vi "Set Begin.vi"(8 "error in (no error)":errorcluster, 10 "Begin":refnum<class "Data.lvclass">, 11 "Range in":refnum<class "Range.lvclass">) -> (0 "error out":errorcluster, 3 "Range out":refnum<class "Range.lvclass">)   [LabVIEW 2015, in "MDSplus.lvlib" / "Range.lvclass"]
uses:
  Range.lvclass
  Data.lvclass
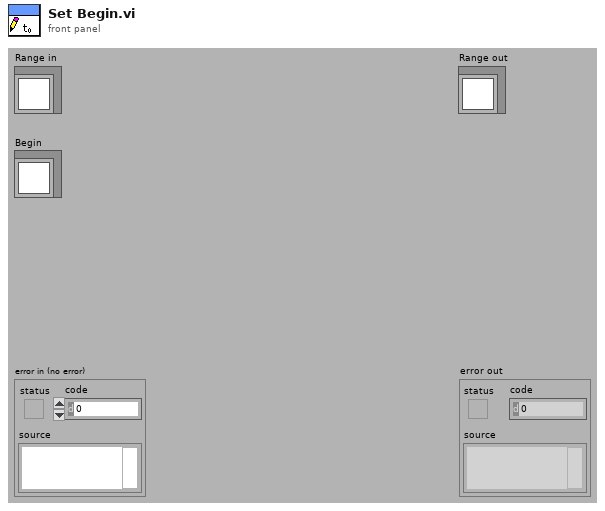
[diagram p1: front panel]
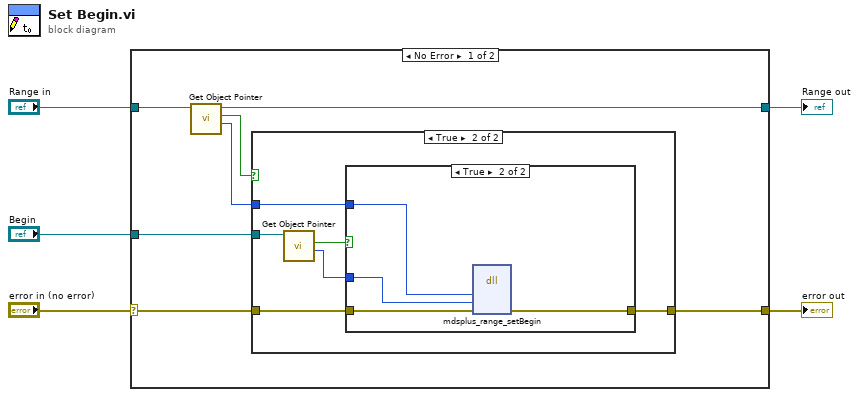
[diagram p0: block diagram]
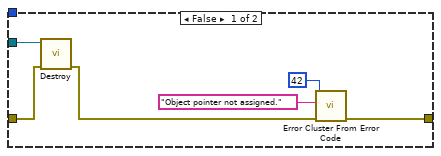
[diagram p2: hidden frame]
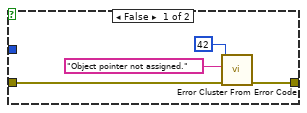
[diagram p3: hidden frame]
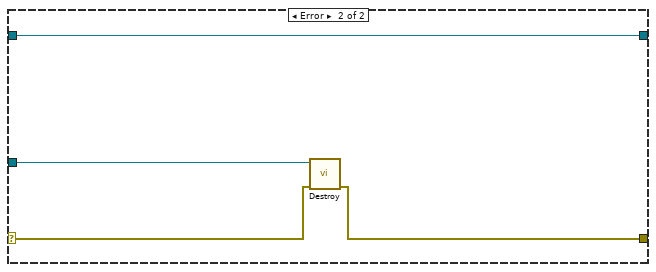
[diagram p4: hidden frame]
diagram:
  n1 = case shown="No Error" "error in (no error)" {
    selector: "error in (no error)" -> [w8 w34]
    tunnel: [w7 w33] -> w4
    tunnel: [w6 w36] -> w2
    tunnel: "Range in" -> [w12 w36]
    tunnel: "Begin" -> [w11 w35]
    frame No Error {
      n2 = call-dynamic "Get Object Pointer.vi"("Data in"=w12) -> ("Object Pointer"=w9:i64, "Assigned object pointer?"=w10:bool, "Data out"=w6:refnum<class "Range.lvclass">)  [unwired: 8 in]
      n3 = case shown="True" w10 {
        tunnel: w11 -> [w15 w24]
        tunnel: w9 -> [_ w21]
        tunnel: w8 -> [w14 w20]
        tunnel: [w16 w19] -> w7
        frame False {
          n4 = call-dynamic "Destroy.vi"("error in (no error)"=w14, "Data in"=w15) -> ("error out"=w13:errorcluster)  [unwired: 9 in]
          n5 = call <vilib>:"Error Cluster From Error Code.vi"("error in (no error)"=w13, "error message (\"\")"="Object pointer not assigned." ("error message (\"\")"), "error code (0)"=42) -> ("error out"=w16:errorcluster)  [unwired: 6 in]
        }
        frame True {
          n6 = call-dynamic "Get Object Pointer.vi"("Data in"=w24) -> ("Object Pointer"=w22:i64, "Assigned object pointer?"=w23:bool)  [unwired: 8 in, 1 out]
          n7 = case shown="True" w23 {
            tunnel: w22 -> [_ w31]
            tunnel: w21 -> [_ w32]
            tunnel: w20 -> [w26 w30]
            tunnel: [w25 w29] -> w19
            frame False {
              n8 = call <vilib>:"Error Cluster From Error Code.vi"("error in (no error)"=w26, "error message (\"\")"="Object pointer not assigned." ("error message (\"\")"), "error code (0)"=42) -> ("error out"=w25:errorcluster)  [unwired: 6 in]
            }
            frame True {
              n9 = dll-call lib="MDSobjectsLVShr" fn="mdsplus_range_setBegin"("lvRangePtr"=w32, "lvDataPtrIn"=w31, "error"=w30) -> ("error"=w29:errorcluster)  [unwired: 6 in, 2 out]
            }
          }
        }
      }
    }
    frame Error {
      n10 = call-dynamic "Destroy.vi"("error in (no error)"=w34, "Data in"=w35) -> ("error out"=w33:errorcluster)  [unwired: 9 in]
    }
  }
  "error out" <- w4
  "Range out" <- w2
